vi "Wait On Occurrence Wrapper.vi"(8 "error in":errorcluster, 10 "ms timeout (-1)":i32=-1, 11 "occurrence in":refnum<k4>) -> (0 "error out":errorcluster)   [LabVIEW 2019, in "grpc-lvsupport.lvlib"]
uses:
  grpc-lvsupport.lvlib
  TranslateGrpcError.vi
  <vilib>/Utility/error.llb/Error Cluster From Error Code.vi
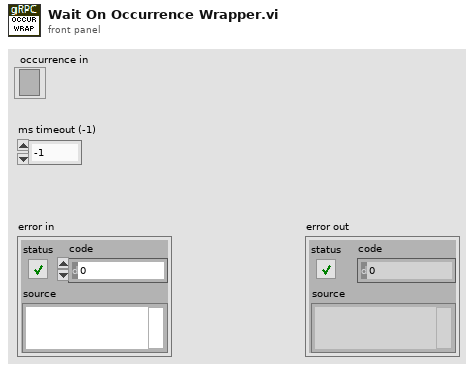
[diagram p1: front panel]
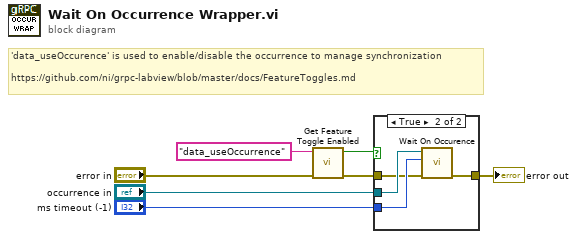
[diagram p0: block diagram]
diagram:
  # "'data_useOccurence' is used to enable/disable the occurrence to manage synchronization\n\nhttps://github.com/ni/grpc-labview/blob/master/docs/FeatureToggles.md"
  n1 = call "Get Feature Toggle Enabled.vi"("error in"="error in", "Feature Name"="data_useOccurrence" ("key")) -> ("error out"=w2:errorcluster, "Feature Enabled?"=w1:bool)  [unwired: 8 in]
  n2 = case shown="True" w1 {
    tunnel: "occurrence in" -> [_ w12]
    tunnel: "ms timeout (-1)" -> [_ w11]
    tunnel: w2 -> [w8 w10]
    tunnel: [w8 w9] -> w5
    frame False {
    }
    frame True {
      n3 = call "Wait On Occurence.vi"("error in"=w10, "ms timeout (-1)"=w11, "occurrence in"=w12) -> ("error out"=w9:errorcluster)  [unwired: 8 in]
    }
  }
  "error out" <- w5
